vi "ExecuteStep.vi"(0 "reference in":refnum<class "Stand.lvclass">, 11 "error in (no error)":errorcluster) -> (4 "reference out":refnum<class "Stand.lvclass">, 15 "error out":errorcluster)   [LabVIEW 2019, in "Stand.lvclass"]
uses:
  Stand.lvclass
  C:/Users/ANENKOV_V1/Desktop/SRC_H400/src/src/Device_class/Device.lvclass
  Stand.lvclass/Stand.ctl
  TypeDef/Direction.ctl
  TypeDef/ExecuteStepState.ctl
  AI_class/AI.lvclass/AI.ctl
  AnalogComparator_class/AnalogComparator.lvclass/AnalogComparator.ctl
  FPGA/TypeDef/AI index.ctl
  Device_class/Device.lvclass/Device.ctl
  NeedleValve_class/Cmd.ctl
  Valve Mode.ctl
  d900ba76-673b-43eb-b747-4a40eb4a2de0.vi
  Haskel Fast Forward.vi
  Set Hi Press.vi/29706e3b-acf2-4be0-8e3a-420f003c1de5.vi
  AnalogComparator_class/GetStatus.vi
  Valve State Mode.vi
  subvis/FastForward.vi
  Get U max Haskel.vi
  Get Accuracy.vi
  Valve State Mode.vi/810e184e-eeb6-4027-a8ae-1422f3ce3d45.vi
  Valve State Mode.vi/57bd4a65-f3dc-44f5-8d68-677c2a197570.vi
  Valve State Mode.vi/03b2f9e4-fceb-4725-9b90-3fd10082a088.vi
  Valve State Mode.vi/3d0d09bd-48e8-482f-b1e2-a36b2bb65234.vi
  Valve State Mode.vi/33d3f26a-dc4a-4f56-bf0a-61d04c5d7434.vi
  Valve State Mode.vi/52af9d47-24d1-4057-80bf-8d93bfb3d17d.vi
  Valve State Mode.vi/094228cb-a119-423c-9af8-5a16f059a318.vi
  Valve State Mode.vi/bf5ad1e6-a0ae-4579-ad74-ca8f304cb7cf.vi
  Valve State Mode.vi/eb4d2b76-f0f0-4e1d-bda0-609c5f37b4e7.vi
  Global/Global Constant.vi
  Const All Valve.vi
  <vilib>/addons/_JKI.lib/FPGA_Basic_Components/Counter JKI_FPGA.vi
  <vilib>/addons/_JKI.lib/FPGA_Basic_Components/Counter_32bit JKI_FPGA.vi
  FPGA_API_class/FPGA API.lvclass
  AI_class/AI.lvclass
  NeedleValve_class/NeedleValve.lvclass
  Device_class/Device.lvclass
panel:
  in  "init":bool
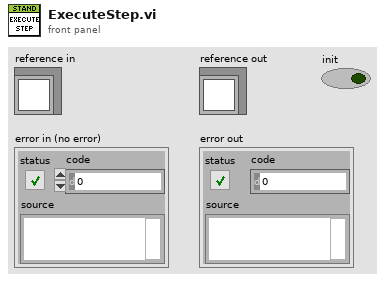
[diagram p1: front panel]
types:
  T1 = typedef "ExecuteStepState.ctl" = enum16{"Init", "Set: Backpressure ", "Preload: HI", "Set: HI", "Maintenance: HI", "Down: Pressure", "BLOCK"}
  T2 = typedef "Direction.ctl" = enum8{"DUT", "Chamber"}
  T3 = typedef "NeedleValve.lvclass/Cmd.ctl" = enum16{"Open", "Close", "Stop"}
  T4 = typedef "Valve Mode.ctl" = enum16{"Filling DUT", "Filling Chamber", "Pump Pressure DUT", "Pump Pressure Chamber", "Haskel Pressure DUT", "Haskel Pressure Chamber", "Slow Release DUT", "Slow Release Chamber", "Fast Release DUT", "Fast Release Chamber", "Fast Release DUT and Chamber", "Leak Pressure DUT", "Leak Pressure Chamber", "Back Pressure DUT", "Back Pressure Chamber", "Fully Closed", "Drain", "Block DUT", "Block Chamber"}
  T5 = typedef "SP_TYPE.ctl" = enum16{"ERROR", "ZIRO", "BASE", "SP"}
  T6 = typedef "AI index.ctl" = u8
  T7 = typedef "AI_Data.ctl" = cluster{"Stat Data":T8, "OutOfRangeMax":bool, "OutOfRangeMin":bool, "HIHI":bool, "HI":bool, "LO":bool, "LOLO":bool}
  T8 = typedef "AI Statistics Data.ctl" = cluster{"raw mean":dbl, "scl mean":dbl, "raw mean 1Hz":dbl, "scl mean 1Hz":dbl}
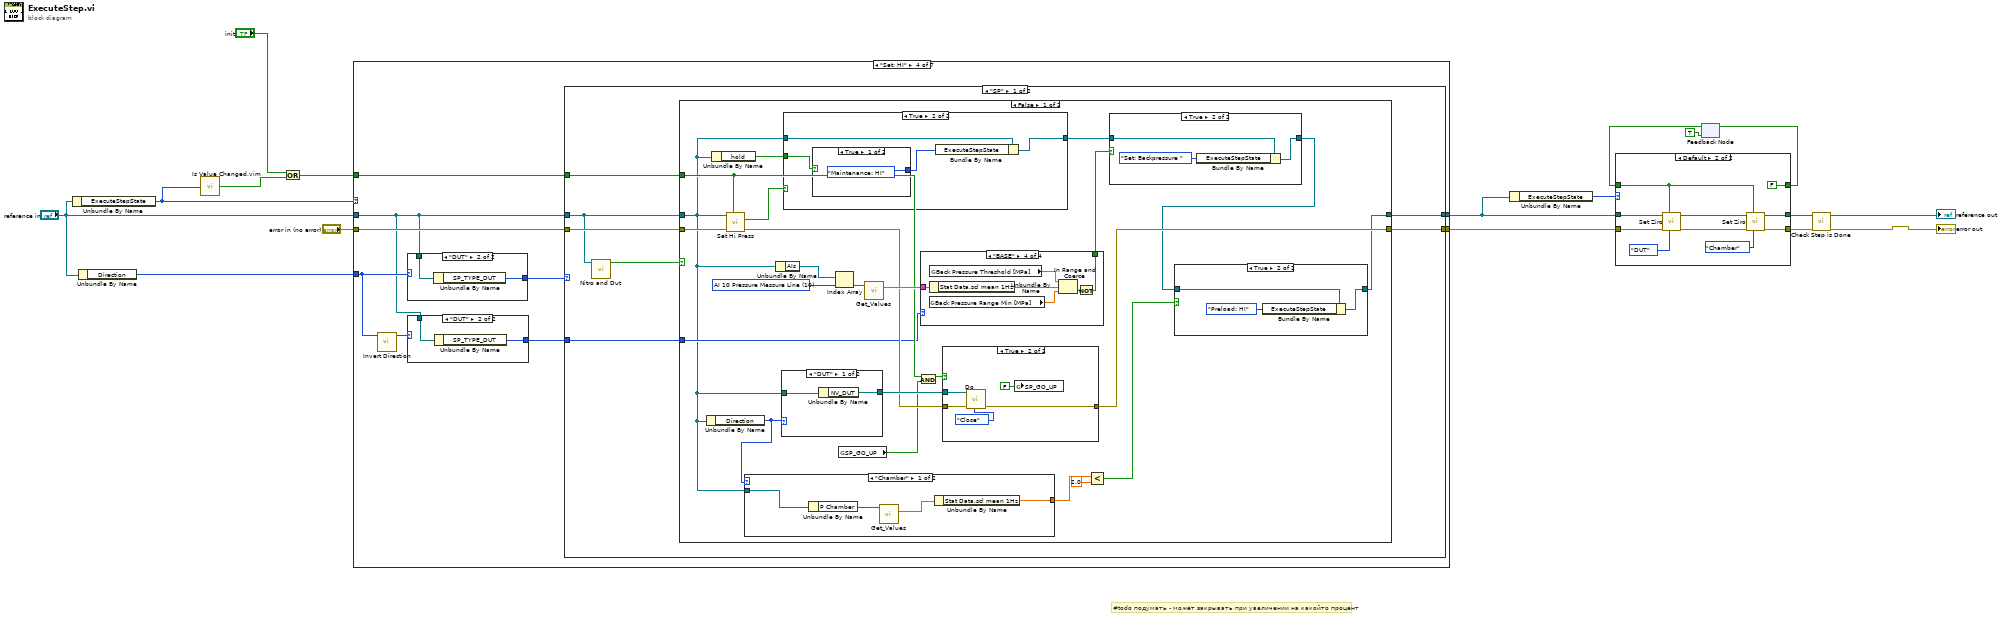
[diagram p0: block diagram]
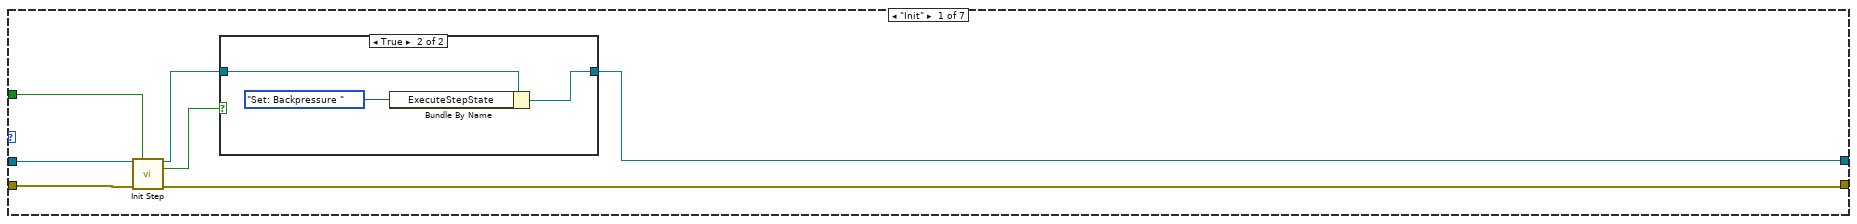
[diagram p2: hidden frame]
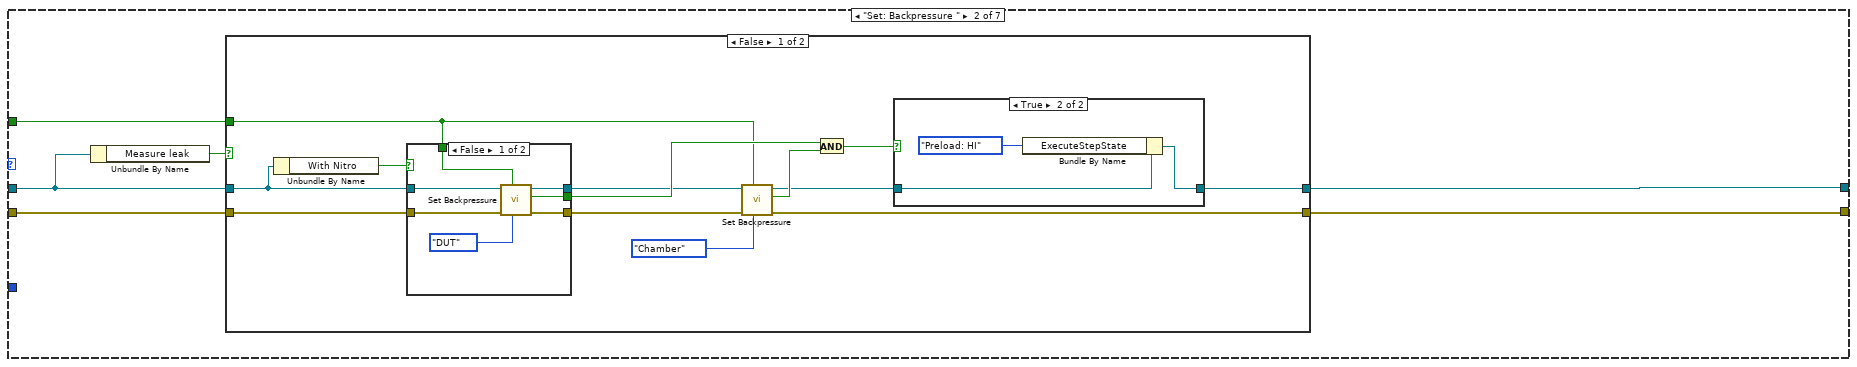
[diagram p4: hidden frame]
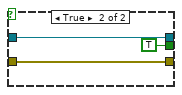
[diagram p5: hidden frame]
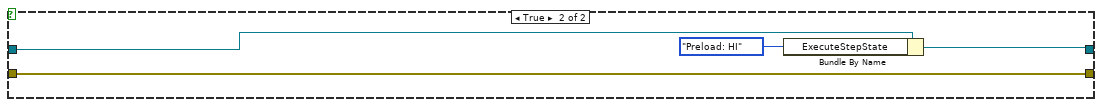
[diagram p7: hidden frame]
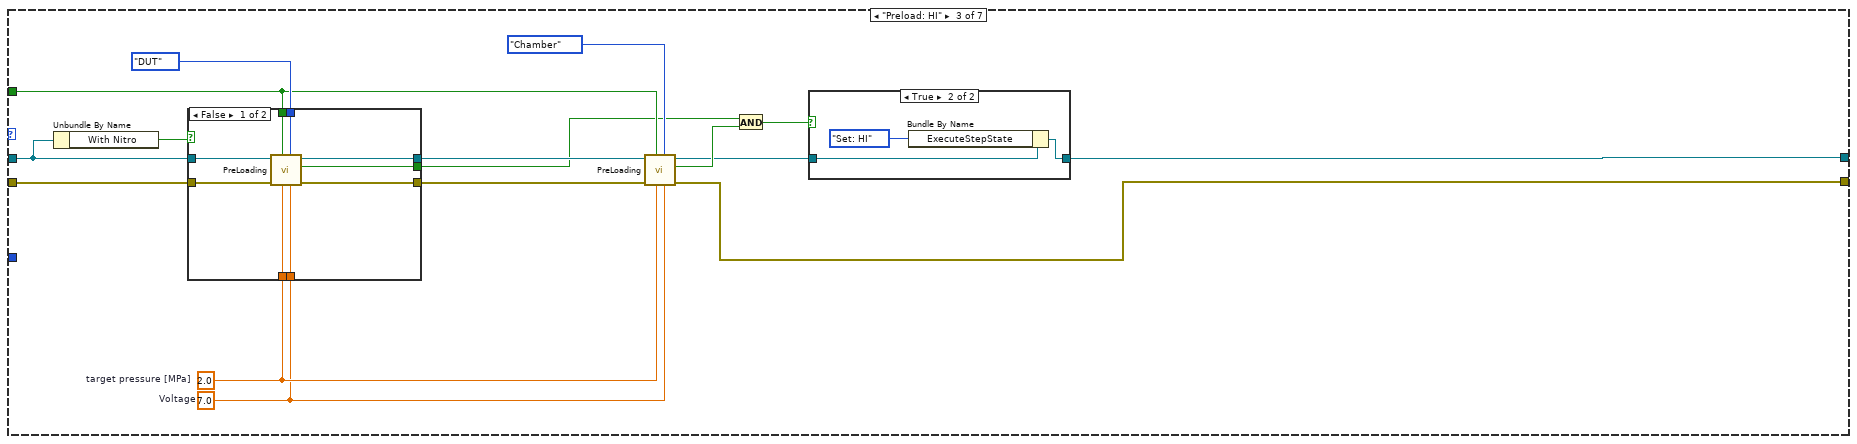
[diagram p8: hidden frame]
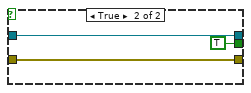
[diagram p9: hidden frame]
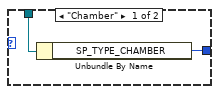
[diagram p11: hidden frame]
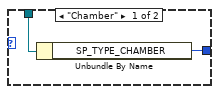
[diagram p12: hidden frame]
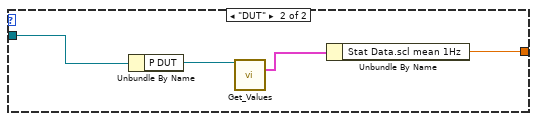
[diagram p13: hidden frame]
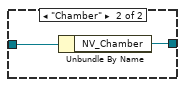
[diagram p18: hidden frame]
diagram:
  # "#todo подумать - может закрывать при увеличении на какойто процент"
  n1 = Unbundle By Name("reference in") -> ("ExecuteStepState"=w15:T1)
  n2 = Unbundle By Name("reference in") -> ("Direction"=w7:T2)
  n3 = call "Is Value Changed.vim"("value"=w15) -> ("changed or first call?"=w14:bool)
  n4 = Or(x="init", y=w14) -> (x .or. y?=w16:bool)
  n5 = case shown="\"Set: HI\"" w15 {
    tunnel: [w18 w33 w80 w105 w196 w234 w281] -> w10
    tunnel: "reference in" -> [w23 w30 w67 w99 w193 w232 w278]
    tunnel: "error in (no error)" -> [w24 w34 w81 w106 w198 w236 w284]
    tunnel: [w22 w31 w68 w104 w197 w235 w282] -> w13
    tunnel: w16 -> [w21 w32 w73 w103 w199 w237 w283]
    tunnel: w7 -> [_ _ _ w101 w195 w230 w280]
    frame "Init" {
      n6 = call "Init Step.vi"("reference in"=w23, "init"=w21, "error in (no error)"=w24) -> ("reference out"=w20:refnum<class "Stand.lvclass">, "done"=w19:bool, "error out"=w22:errorcluster)  [unwired: 10 in]
      n7 = case shown="True" w19 {
        tunnel: [w25 w26] -> w18
        tunnel: w20 -> [w25 w28]
        frame False {
        }
        frame True {
          n8 = Bundle By Name(cluster=w28, "ExecuteStepState"=ExecuteStepState."Set: Backpressure ") -> (w26:refnum<class "Stand.lvclass">)
        }
      }
    }
    frame "Set: Backpressure " {
      n9 = Unbundle By Name(w30) -> ("Measure leak"=w29:bool)
      n10 = case shown="False" w29 {
        tunnel: w34 -> [w47 w65]
        tunnel: [w45 w62] -> w33
        tunnel: w32 -> [w43 _]
        tunnel: [w37 w65] -> w31
        tunnel: w30 -> [w36 w63]
        frame False {
          n11 = Unbundle By Name(w36) -> ("With Nitro"=w35:bool)
          n12 = case shown="False" w35 {
            tunnel: w47 -> [w54 w56]
            tunnel: [w53 TRUE ("done")] -> w46
            tunnel: [w51 w57] -> w44
            tunnel: w43 -> [w50 _]
            tunnel: [w49 w56] -> w42
            tunnel: w36 -> [w48 w57]
            frame False {
              n13 = call "Set Backpressure.vi"("Direction"=Direction."DUT", "init"=w50, "error in (no error)"=w54, "Stand in"=w48) -> ("error out"=w49:errorcluster, "done"=w53:bool, "Stand out"=w51:refnum<class "Stand.lvclass">)  [unwired: 5 in]
            }
            frame True {
            }
          }
          n14 = call "Set Backpressure.vi"("Direction"=Direction."Chamber", "init"=w43, "error in (no error)"=w42, "Stand in"=w44) -> ("error out"=w37:errorcluster, "done"=w39:bool, "Stand out"=w38:refnum<class "Stand.lvclass">)  [unwired: 5 in]
          n15 = And(x=w46, y=w39) -> (x .and. y?=w40:bool)
          n16 = case shown="True" w40 {
            tunnel: [w58 w59] -> w45
            tunnel: w38 -> [w58 w61]
            frame False {
            }
            frame True {
              n17 = Bundle By Name(cluster=w61, "ExecuteStepState"=ExecuteStepState."Preload: HI") -> (w59:refnum<class "Stand.lvclass">)
            }
          }
        }
        frame True {
          n18 = Bundle By Name(cluster=w63, "ExecuteStepState"=ExecuteStepState."Preload: HI") -> (w62:refnum<class "Stand.lvclass">)
        }
      }
    }
    frame "Preload: HI" {
      w76 = 7.0  # Voltage
      w77 = 2.0  # target pressure [MPa]
      n19 = Unbundle By Name(w67) -> ("With Nitro"=w66:bool)
      n20 = case shown="False" w66 {
        tunnel: w81 -> [w90 w91]
        tunnel: Direction."DUT" ("Direction") -> [w89 _]
        tunnel: w77 -> [w88 _]
        tunnel: w76 -> [w87 _]
        tunnel: [w86 w93] -> w75
        tunnel: [w85 w91] -> w74
        tunnel: w73 -> [w84 _]
        tunnel: [w83 TRUE ("done")] -> w71
        tunnel: w67 -> [w82 w93]
        frame False {
          n21 = call "PreLoading.vi"("Voltage"=w87, "Direction"=w89, "target pressure [MPa]"=w88, "init"=w84, "error in (no error)"=w90, "Stand in"=w82) -> ("error out"=w85:errorcluster, "done"=w83:bool, "Stand out"=w86:refnum<class "Stand.lvclass">)  [unwired: 3 in]
        }
        frame True {
        }
      }
      n22 = call "PreLoading.vi"("Voltage"=w76, "Direction"=Direction."Chamber", "target pressure [MPa]"=w77, "init"=w73, "error in (no error)"=w74, "Stand in"=w75) -> ("error out"=w68:errorcluster, "done"=w72:bool, "Stand out"=w70:refnum<class "Stand.lvclass">)  [unwired: 3 in]
      n23 = And(x=w71, y=w72) -> (x .and. y?=w69:bool)
      n24 = case shown="True" w69 {
        tunnel: [w94 w96] -> w80
        tunnel: w70 -> [w94 w95]
        frame False {
        }
        frame True {
          n25 = Bundle By Name(cluster=w95, "ExecuteStepState"=ExecuteStepState."Set: HI") -> (w96:refnum<class "Stand.lvclass">)
        }
      }
    }
    frame "Set: HI" {
      n26 = call "Invert Direction.vi"("Direction"=w101) -> ("invert Direction"=w100:T2)  [unwired: 10 in]
      n27 = case shown="\"DUT\"" w101 {
        tunnel: w99 -> [w112 w114]
        tunnel: [w111 w113] -> w102
        frame "Chamber" {
          n28 = Unbundle By Name(w112) -> ("SP_TYPE_CHAMBER"=w111:T5)
        }
        frame "DUT" {
          n29 = Unbundle By Name(w114) -> ("SP_TYPE_DUT"=w113:T5)
        }
      }
      n30 = case shown="\"DUT\"" w100 {
        tunnel: w99 -> [w108 w110]
        tunnel: [w107 w109] -> w98
        frame "Chamber" {
          n31 = Unbundle By Name(w108) -> ("SP_TYPE_CHAMBER"=w107:T5)
        }
        frame "DUT" {
          n32 = Unbundle By Name(w110) -> ("SP_TYPE_DUT"=w109:T5)
        }
      }
      n33 = case shown="\"SP\"" w102 {
        tunnel: w106 -> [w121 w191]
        tunnel: [w120 w190] -> w105
        tunnel: w99 -> [w116 w188]
        tunnel: [w119 w191] -> w104
        tunnel: w103 -> [w118 _]
        tunnel: w98 -> [w117 _]
        frame "SP" {
          n34 = call "Nitro and Dut.vi"("Stand in"=w116) -> ("nitro and dut"=w115:bool)  [unwired: 10 in]
          n35 = case shown="False" w115 {
            tunnel: w121 -> [w144 w187]
            tunnel: [w127 w184] -> w120
            tunnel: [w136 w187] -> w119
            tunnel: w118 -> [w135 _]
            tunnel: w117 -> [w132 _]
            tunnel: w116 -> [w126 w185]
            frame False {
              w141 = T6 10 items=["AI 0 Cooling Station Level", "AI 1 Cooling Station Temp", "AI 2 Oil Supply Level", "AI 3 Oil Supply Temp", "AI 4 ", "AI 5 Pressure Haskel", "AI 6 Pressure DUT", "AI 7 Pressure Chamber", "AI 8 Pressure Air inlet", "AI 9 Pressure Air outlet", "AI 10 Pressure Messure Line", "AI 11 DUT 2", "AI 12 Chamber 2"] ("AI index")
              n36 = Unbundle By Name(w126) -> ("Direction"=w125:T2)
              n37 = Unbundle By Name(w126) -> ("hold"=w129:bool)
              n38 = call "Set Hi Press.vi"("init"=w135, "error in (no error)"=w144, "Stand in"=w126) -> ("error out"=w133:errorcluster, "Done"=w143:bool)  [unwired: 7 in]
              n39 = case shown="\"Chamber\"" w125 {
                tunnel: w126 -> [w147 w151]
                tunnel: [w145 w149] -> w124
                frame "Chamber" {
                  n40 = Unbundle By Name(w147) -> ("P Chamber"=w146:refnum<class "AI.lvclass">)
                  n41 = call "Get_Values.vi"("reference in"=w146) -> ("Data"=w148:T7)  [unwired: 14 in]
                  n42 = Unbundle By Name(w148) -> ("Stat Data.scl mean 1Hz"=w145:dbl)
                }
                frame "DUT" {
                  n43 = Unbundle By Name(w151) -> ("P DUT"=w150:refnum<class "AI.lvclass">)
                  n44 = call "Get_Values.vi"("reference in"=w150) -> ("Data"=w152:T7)  [unwired: 14 in]
                  n45 = Unbundle By Name(w152) -> ("Stat Data.scl mean 1Hz"=w149:dbl)
                }
              }
              n46 = Unbundle By Name(w126) -> ("AIs"=w142:refnum<class "AI.lvclass">[])
              n47 = case shown="\"DUT\"" w125 {
                tunnel: [w164 w166] -> w137
                tunnel: w126 -> [w163 w165]
                frame "DUT" {
                  n48 = Unbundle By Name(w163) -> ("NV_DUT"=w164:refnum<class "NeedleValve.lvclass">)
                }
                frame "Chamber" {
                  n49 = Unbundle By Name(w165) -> ("NV_Chamber"=w166:refnum<class "NeedleValve.lvclass">)
                }
              }
              n50 = case shown="True" w143 {
                tunnel: [w177 w180] -> w138
                tunnel: w126 -> [w177 w179]
                tunnel: w129 -> [_ w178]
                frame False {
                }
                frame True {
                  n51 = case shown="True" w178 {
                    tunnel: [ExecuteStepState."Maintenance: HI" ("ExecuteStepState") ExecuteStepState."BLOCK" ("ExecuteStepState")] -> w181
                    frame True {
                    }
                    frame False {
                    }
                  }
                  n52 = Bundle By Name(cluster=w179, "ExecuteStepState"=w181) -> (w180:refnum<class "Stand.lvclass">)
                }
              }
              n53 = Index Array(array=w142, index=w141) -> (element=w140:refnum<class "AI.lvclass">)
              n54 = global read "Global Constant.vi" "SP_GO_UP"() -> (w130:bool)
              n55 = call "Get_Values.vi"("reference in"=w140) -> ("Data"=w139:T7)  [unwired: 14 in]
              n56 = And(x=w135, y=w130) -> (x .and. y?=w131:bool)
              n57 = case shown="\"BASE\"" w132 {
                tunnel: w139 -> [_ _ _ w162]
                tunnel: [_ _ _ w159] -> w134
                frame "ERROR" {
                }
                frame "ZIRO" {
                }
                frame "SP" {
                }
                frame "BASE" {
                  n58 = Unbundle By Name(w162) -> ("Stat Data.scl mean 1Hz"=w158:dbl)
                  n59 = global read "Global Constant.vi" "Back Pressure Range Min [MPa]"() -> (w161:dbl)
                  n60 = global read "Global Constant.vi" "Back Pressure Threshold [MPa]"() -> (w157:dbl)
                  n61 = In Range and Coerce(upper limit=w157, x=w158, lower limit=w161) -> (In Range?=w160:bool)  [unwired: 1 out]
                  n62 = Not(x=w160) -> (.not. x?=w159:bool)
                }
              }
              n63 = case shown="True" w131 {
                tunnel: [w167 w172] -> w136
                tunnel: w137 -> [_ w170]
                tunnel: w133 -> [w167 w169]
                frame False {
                }
                frame True {
                  n64 = call "Do.vi"("Cmd"=Cmd."Close", "error in (no error)"=w169, "NeedleValve in"=w170) -> ("error out"=w172:errorcluster)  [unwired: 7 in, 1 out]
                  n65 = global write "Global Constant.vi" "SP_GO_UP"(FALSE ("SP_GO_UP")) -> ()
                }
              }
              n66 = Less?(x=w124, y=2.0) -> (x < y?=w122:bool)
              n67 = case shown="True" w134 {
                tunnel: w138 -> [w173 w176]
                tunnel: [w173 w175] -> w128
                frame False {
                }
                frame True {
                  n68 = Bundle By Name(cluster=w176, "ExecuteStepState"=ExecuteStepState."Set: Backpressure " ("Data.ExecuteStepState")) -> (w175:refnum<class "Stand.lvclass">)
                }
              }
              n69 = case shown="True" w122 {
                tunnel: w128 -> [w153 w156]
                tunnel: [w153 w155] -> w127
                frame False {
                }
                frame True {
                  n70 = Bundle By Name(cluster=w156, "ExecuteStepState"=ExecuteStepState."Preload: HI" ("Data.ExecuteStepState")) -> (w155:refnum<class "Stand.lvclass">)
                }
              }
            }
            frame True {
              n71 = Bundle By Name(cluster=w185, "ExecuteStepState"=ExecuteStepState."Set: Backpressure " ("Data.ExecuteStepState")) -> (w184:refnum<class "Stand.lvclass">)
            }
          }
        }
        frame Default {
          n72 = Bundle By Name(cluster=w188, "ExecuteStepState"=ExecuteStepState."Set: Backpressure " ("Data.ExecuteStepState")) -> (w190:refnum<class "Stand.lvclass">)
        }
      }
    }
    frame "Maintenance: HI" {
      n73 = case shown="\"DUT\"" w195 {
        tunnel: w193 -> [w227 w229]
        tunnel: [w226 w228] -> w194
        frame "Chamber" {
          n74 = Unbundle By Name(w227) -> ("SP_TYPE_CHAMBER"=w226:T5)
        }
        frame "DUT" {
          n75 = Unbundle By Name(w229) -> ("SP_TYPE_DUT"=w228:T5)
        }
      }
      n76 = call "Nitro and Dut.vi"("Stand in"=w193) -> ("nitro and dut"=w192:bool)  [unwired: 10 in]
      n77 = case shown="False" w192 {
        tunnel: w199 -> [w205 _]
        tunnel: w198 -> [w204 w223]
        tunnel: [w203 w223] -> w197
        tunnel: [w202 w222] -> w196
        tunnel: w194 -> [w201 _]
        tunnel: w193 -> [w200 w224]
        frame False {
          n78 = case shown="\"SP\"" w201 {
            tunnel: w205 -> [_ w215]
            tunnel: w204 -> [w208 w217]
            tunnel: [w208 w216] -> w203
            tunnel: [w207 w210] -> w202
            tunnel: w200 -> [w209 w213]
            frame Default {
              n79 = Bundle By Name(cluster=w209, "ExecuteStepState"=ExecuteStepState."Set: Backpressure " ("Data.ExecuteStepState")) -> (w207:refnum<class "Stand.lvclass">)
            }
            frame "SP" {
              n80 = call "Set Hi Press.vi"("init"=w215, "error in (no error)"=w217, "Stand in"=w213) -> ("error out"=w214:errorcluster)  [unwired: 7 in, 1 out]
              n81 = call "Check Range Hi Press.vi"("reference in"=w213, "init"=w215, "error in (no error)"=w214) -> ("reference out"=w211:refnum<class "Stand.lvclass">, "error out"=w216:errorcluster)  [unwired: 11 in]
              n82 = Unbundle By Name(w213) -> ("hold"=w212:bool)
              n83 = case shown="False" w212 {
                tunnel: w211 -> [w220 w221]
                tunnel: [w218 w221] -> w210
                frame False {
                  n84 = Bundle By Name(cluster=w220, "ExecuteStepState"=ExecuteStepState."BLOCK" ("Data.ExecuteStepState")) -> (w218:refnum<class "Stand.lvclass">)
                }
                frame True {
                }
              }
            }
          }
        }
        frame True {
          n85 = Bundle By Name(cluster=w224, "ExecuteStepState"=ExecuteStepState."Set: Backpressure " ("Data.ExecuteStepState")) -> (w222:refnum<class "Stand.lvclass">)
        }
      }
    }
    frame "BLOCK" {
      n86 = case shown="\"DUT\"" w230 {
        tunnel: w232 -> [w274 w276]
        tunnel: [w273 w275] -> w233
        frame "Chamber" {
          n87 = Unbundle By Name(w274) -> ("SP_TYPE_CHAMBER"=w273:T5)
        }
        frame "DUT" {
          n88 = Unbundle By Name(w276) -> ("SP_TYPE_DUT"=w275:T5)
        }
      }
      n89 = call "Nitro and Dut.vi"("Stand in"=w232) -> ("nitro and dut"=w231:bool)  [unwired: 10 in]
      n90 = case shown="False" w231 {
        tunnel: w237 -> [w244 _]
        tunnel: w236 -> [w243 w270]
        tunnel: [w242 w270] -> w235
        tunnel: [w241 w269] -> w234
        tunnel: w233 -> [w240 _]
        tunnel: w232 -> [w239 w271]
        tunnel: w230 -> [w238 _]
        frame False {
          n91 = case shown="\"SP\"" w240 {
            tunnel: w244 -> [_ w255]
            tunnel: w243 -> [w247 w260]
            tunnel: [w247 w262] -> w242
            tunnel: [w246 w250] -> w241
            tunnel: w239 -> [w248 w258]
            tunnel: w238 -> [_ w253]
            frame Default {
              n92 = Bundle By Name(cluster=w248, "ExecuteStepState"=ExecuteStepState."Set: Backpressure " ("Data.ExecuteStepState")) -> (w246:refnum<class "Stand.lvclass">)
            }
            frame "SP" {
              n93 = case shown="\"Chamber\"" w253 {
                tunnel: [Valve_Mode."Block Chamber" ("Valve DIR") Valve_Mode."Block DUT" ("Valve DIR")] -> w254
                frame "Chamber" {
                }
                frame "DUT" {
                }
              }
              n94 = call "GetFPGA.vi"("Device in"=w258) -> ("FPGA API.lvclass"=w261:refnum<class "FPGA API.lvclass">)  [unwired: 10 in]
              n95 = call-dynamic "SetHasckelAO.vi"("FPGA API in"=w261, "Haskel in"=0.0, "error in (no error)"=w260) -> ("error out"=w257:errorcluster)  [unwired: 11 in, 1 out]
              n96 = call "Set Valve Mode.vi"("time after close"=u32 0, "Valve DIR"=w254, "init"=w255, "error in (no error)"=w257, "Stand in"=w258) -> ("error out"=w256:errorcluster)  [unwired: 5 in, 1 out]
              n97 = call "Check Range Hi Press.vi"("reference in"=w258, "init"=w255, "error in (no error)"=w256) -> ("reference out"=w249:refnum<class "Stand.lvclass">, "error out"=w262:errorcluster)  [unwired: 11 in]
              n98 = Unbundle By Name(w249) -> ("hold"=w251:bool)
              n99 = case shown="True" w251 {
                tunnel: w249 -> [w263 w266]
                tunnel: [w263 w264] -> w250
                frame False {
                }
                frame True {
                  n100 = Bundle By Name(cluster=w266, "ExecuteStepState"=ExecuteStepState."Maintenance: HI" ("Data.ExecuteStepState")) -> (w264:refnum<class "Stand.lvclass">)
                }
              }
            }
          }
        }
        frame True {
          n101 = Bundle By Name(cluster=w271, "ExecuteStepState"=ExecuteStepState."Set: Backpressure " ("Data.ExecuteStepState")) -> (w269:refnum<class "Stand.lvclass">)
        }
      }
    }
    frame "Down: Pressure" {
      n102 = case shown="\"DUT\"" w280 {
        tunnel: w278 -> [w310 w312]
        tunnel: [w309 w311] -> w279
        frame "Chamber" {
          n103 = Unbundle By Name(w310) -> ("SP_TYPE_CHAMBER"=w309:T5)
        }
        frame "DUT" {
          n104 = Unbundle By Name(w312) -> ("SP_TYPE_DUT"=w311:T5)
        }
      }
      n105 = call "Nitro and Dut.vi"("Stand in"=w278) -> ("nitro and dut"=w277:bool)  [unwired: 10 in]
      n106 = case shown="False" w277 {
        tunnel: w284 -> [w290 w308]
        tunnel: w283 -> [w289 _]
        tunnel: [w288 w308] -> w282
        tunnel: [w287 w305] -> w281
        tunnel: w279 -> [w286 _]
        tunnel: w278 -> [w285 w306]
        frame False {
          n107 = case shown="\"SP\"" w286 {
            tunnel: w290 -> [w291 w300]
            tunnel: w289 -> [_ w299]
            tunnel: w285 -> [w292 w293]
            tunnel: [w291 w297] -> w288
            tunnel: [w292 w296] -> w287
            frame "ERROR", Default {
            }
            frame "SP" {
              n108 = Unbundle By Name(w293) -> ("Direction"=w298:T2)
              n109 = call "Down Pressure.vi"("Direction"=w298, "init"=w299, "error in (no error)"=w300, "Stand in"=w293) -> ("error out"=w297:errorcluster, "done"=w294:bool, "Stand out"=w295:refnum<class "Stand.lvclass">)  [unwired: 5 in]
              n110 = case shown="True" w294 {
                tunnel: [w301 w303] -> w296
                tunnel: w295 -> [w301 w304]
                frame False {
                }
                frame True {
                  n111 = Bundle By Name(cluster=w304, "ExecuteStepState"=ExecuteStepState."Set: Backpressure " ("Data.ExecuteStepState")) -> (w303:refnum<class "Stand.lvclass">)
                }
              }
            }
          }
        }
        frame True {
          n112 = Bundle By Name(cluster=w306, "ExecuteStepState"=ExecuteStepState."Set: Backpressure " ("Data.ExecuteStepState")) -> (w305:refnum<class "Stand.lvclass">)
        }
      }
    }
  }
  n113 = Unbundle By Name(w10) -> ("ExecuteStepState"=w9:T1)
  n114 = feedback #1(TRUE) -> (w4:bool)
  n115 = case shown="Default" w9 {
    tunnel: w13 -> [w314 w323]
    tunnel: w10 -> [w315 w322]
    tunnel: [w315 w321] -> w12
    tunnel: [w314 w320] -> w11
    tunnel: [TRUE FALSE] -> w6
    tunnel: w4 -> [_ w319]
    frame "Init" {
    }
    frame Default {
      n116 = call "Set Ziro.vi"("Direction"=Direction."DUT", "init"=w319, "error in (no error)"=w323, "Stand in"=w322) -> ("error out"=w324:errorcluster, "Stand out"=w325:refnum<class "Stand.lvclass">)  [unwired: 6 in]
      n117 = call "Set Ziro.vi"("Direction"=Direction."Chamber", "init"=w319, "error in (no error)"=w324, "Stand in"=w325) -> ("error out"=w320:errorcluster, "Stand out"=w321:refnum<class "Stand.lvclass">)  [unwired: 6 in]
    }
  }
  n118 = feedback-in #1(w6) -> ()
  n119 = call "Check Step is Done.vi"("error in (no error)"=w11, "Stand in"=w12) -> ("error out"=→"error out":errorcluster, "Stand out"=→"reference out":refnum<class "Stand.lvclass">)  [unwired: 8 in]
